vi "SignalGenerator.vi"(7 "Signal Output\nControl":enum32{"White Noise", "Harmonic"}(tab), 8 "#s":dbl=41200.0, 9 "Fs":dbl=41200.0, 10 "Hamonic\nParameters":T3={"Waveform Type"=0, "Frequency (Hz)"=10.0, "Amplitude"=0.25} {"Frequency (Hz)" min=5.0 max=350.0 step=10.0 format="%0.2p"; "Waveform Type" items=["Sine Wave", "Triangle Wave", "Square Wave", "Sawtooth Wave"]; "Amplitude" min=0.001 max=0.3 step=0.05 format="%0.2p"}, 11 "White Noise\nParameters":T2={"Seed"=0.0, "Standard Deviation"=2.0, "Reset"=FALSE, "Iterator"=1.0, "Lower Cut-Off"=5.0, "Upper Cut-Off"=350.0} {"Upper Cut-Off" min=5.0 max=350.0 step=10.0; "Lower Cut-Off" min=5.0 max=350.0 step=10.0; "Standard Deviation" min=0.001 max=3.0 step=0.05 format="%0.2p"}) -> (3 "Signal Out":waveform(dbl))   [LabVIEW 2022 SP3]
uses:
  WhiteNoise.ctl
  <vilib>/Analysis/3filter.llb/Filter Passband Type.ctl
  <vilib>/Analysis/3filter.llb/Butterworth Filter (DBL).vi
  <vilib>/measure/NI_MABase.lvlib
  <vilib>/Analysis/NI_AALBase.lvlib
panel:
  # "Filter"
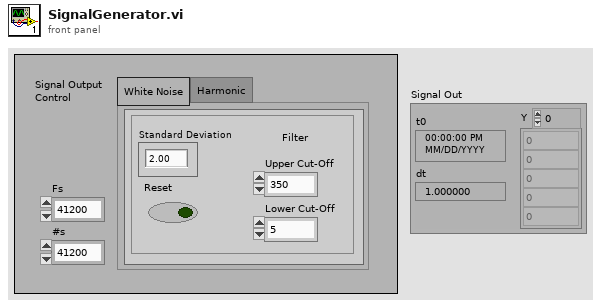
[diagram p1: front panel]
types:
  T1 = typedef "WhiteNoise.ctl" = dbl
  T2 = cluster{"Seed":T1, "Standard Deviation":dbl, "Reset":bool, "Iterator":dbl, "Lower Cut-Off":dbl, "Upper Cut-Off":dbl}
  T3 = cluster{"Waveform Type":u16, "Frequency (Hz)":dbl, "Amplitude":dbl}
  T4 = typedef "NI_AALBase.lvlib/Filter Passband Type.ctl" = enum32{"Lowpass", "Highpass", "Bandpass", "Bandstop"}
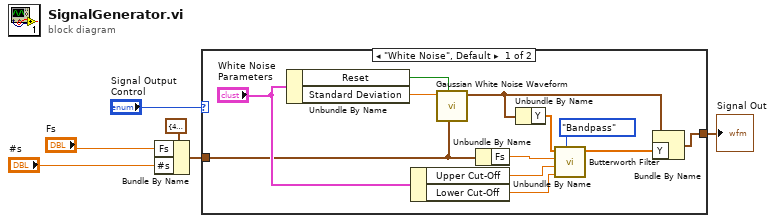
[diagram p0: block diagram]
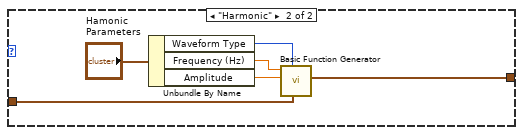
[diagram p2: hidden frame]
diagram:
  n1 = Bundle By Name(cluster=cluster{"Fs":dbl, "#s":dbl} {"Fs"=41200.0, "#s"=41200.0} ("sampling info"), "Fs"="Fs", "#s"="#s") -> (w5:cluster{"Fs":dbl, "#s":dbl})
  n2 = case shown="\"White Noise\", Default" "Signal Output\nControl" {
    tunnel: w5 -> [w13 w23]
    tunnel: [w9 w19] -> w1
    frame "White Noise", Default {
      n3 = Unbundle By Name("White Noise\nParameters") -> ("Reset"=w17:bool, "Standard Deviation"=w18:dbl)
      n4 = Unbundle By Name("White Noise\nParameters") -> ("Upper Cut-Off"=w15:dbl, "Lower Cut-Off"=w14:dbl)
      n5 = call <vilib>:"Gaussian White Noise Waveform.vi"("sampling info"=w13, "reset signal"=w17, "standard deviation"=w18) -> ("signal out"=w8:waveform(dbl))  [unwired: 7 in, 1 out]
      n6 = Unbundle By Name(w13) -> ("Fs"=w12:dbl)
      n7 = Unbundle By Name(w8) -> ("Y"=w7:dbl[])
      n8 = call-poly <vilib>:"Butterworth Filter.vi"("filter type"=Filter_Passband_Type."Bandpass", "low cutoff freq: fl"=w14, "high cutoff freq: fh"=w15, "sampling freq: fs"=w12, "X"=w7) -> ("Filtered X"=w10:dbl[])  [unwired: 3 in, 1 out]
      n9 = Bundle By Name(cluster=w8, "Y"=w10) -> (w9:waveform(dbl))
    }
    frame "Harmonic" {
      n10 = Unbundle By Name("Hamonic\nParameters") -> ("Waveform Type"=w22:u16, "Frequency (Hz)"=w21:dbl, "Amplitude"=w20:dbl)
      n11 = call <vilib>:"Basic Function Generator.vi"("sampling info"=w23, "signal type"=w22, "amplitude"=w20, "frequency"=w21) -> ("signal out"=w19:waveform(dbl))  [unwired: 5 in, 2 out]
    }
  }
  "Signal Out" <- w1
